vi "ProdaNG.Tree.WabcoPart.Add.vi"(7 "Tree":refnum<vi>, 8 "error in (no error)":errorcluster, 10 "WabcoPart":T1) -> (0 "error out":errorcluster, 1 "tag":string)   [LabVIEW 2016]
uses:
  Controls/ProdaNG.WabcoPart.ctl
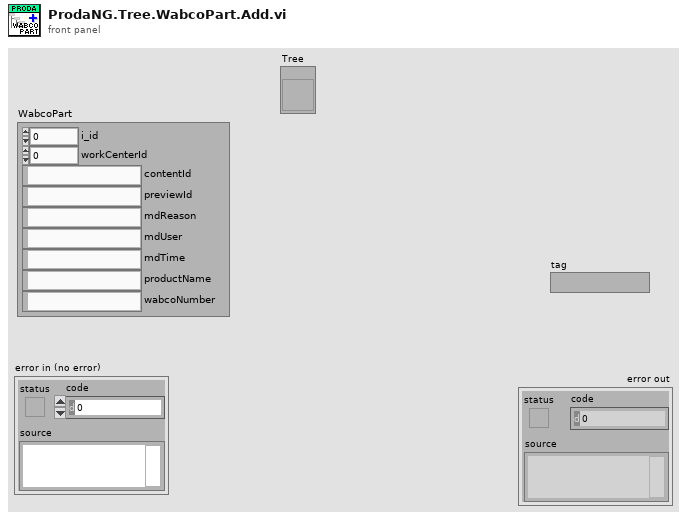
[diagram p1: front panel]
types:
  T1 = typedef "ProdaNG.WabcoPart.ctl" = cluster{"i_id":i32, "workCenterId":i32, "contentId":string, "previewId":string, "mdReason":string, "mdUser":string, "mdTime":string, "productName":string, "wabcoNumber":string}
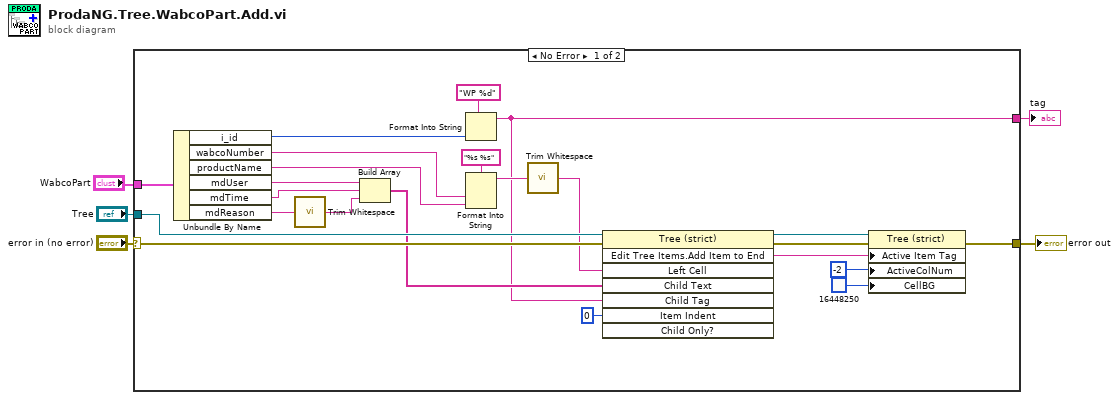
[diagram p0: block diagram]
diagram:
  n1 = case shown="No Error" "error in (no error)" {
    selector: "error in (no error)" -> [w28 w29]
    tunnel: [w15 w29] -> w4
    tunnel: "Tree" -> [w27 _]
    tunnel: "WabcoPart" -> [w26 _]
    tunnel: [w10 _] -> w1
    frame No Error {
      n2 = Unbundle By Name(w26) -> ("i_id"=w24:i32, "wabcoNumber"=w25:string, "productName"=w23:string, "mdUser"=w9:string, "mdTime"=w8:string, "mdReason"=w7:string)
      n3 = call <vilib>:"Trim Whitespace.vi"("string"=w7) -> ("trimmed string"=w6:string)  [unwired: 1 in]
      n4 = Build Array(w9, w8, w6) -> (w21:string[])
      n5 = Format Into String(format string="WP %d", w24) -> (resulting string=w10:string)  [unwired: 2 in, 1 out]
      n6 = Format Into String(format string="%s %s", w25, w23) -> (resulting string=w20:string)  [unwired: 2 in, 1 out]
      n7 = call <vilib>:"Trim Whitespace.vi"("string"=w20) -> ("trimmed string"=w19:string)  [unwired: 1 in]
      n8 = invoke class="Tree (strict)" method="Edit Tree Items.Add Item to End"(reference=w27, error in=w28, "Left Cell"=w19, "Child Text"=w21, "Child Tag"=w10, "Item Indent"=0 ("New Item Indentation")) -> (reference out=w17:refnum<vi>, error out=w16:errorcluster, "Edit Tree Items:Add Item to End"=w11:string)  [unwired: 2 in, 5 out]
      n9 = property class="Tree (strict)"(reference=w17, error in=w16, "Active Item Tag"=w11, "ActiveColNum"=-2 ("Active Cell:Active Column Number"), "CellBG"=u32 16448250) -> (error out=w15:errorcluster)  [unwired: 1 out]
    }
    frame Error {
    }
  }
  "error out" <- w4
  "tag" <- w1
